vi "close.vi"(8 "error in":errorcluster, 11 "Sequencer Module runtime in":refnum<class "Sequencer Module runtime.lvclass">) -> (0 "error out":errorcluster)   [LabVIEW 2015, in "Sequencer Module runtime.lvclass"]
doc: "Provides an interface for terminating a module instance. While this interface performs no operations, a child should close and deallocate any open references or memory."
uses:
  Sequencer Module runtime.lvclass
  Sequencer Module runtime.lvclass/Sequencer Module runtime.ctl
  classes/Result Processor/Execution/ResultProcessor.lvclass
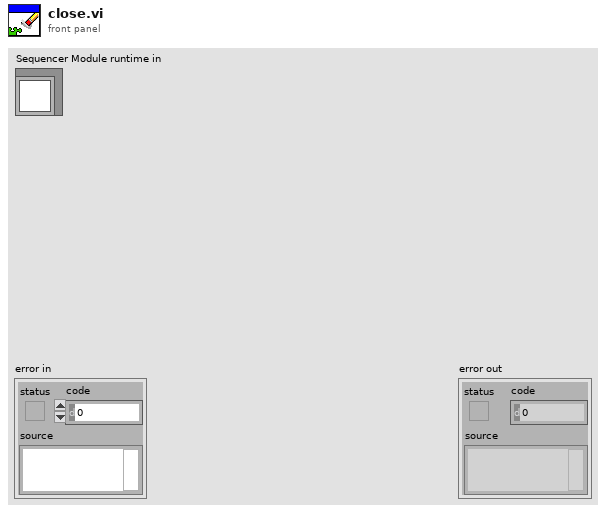
[diagram p1: front panel]
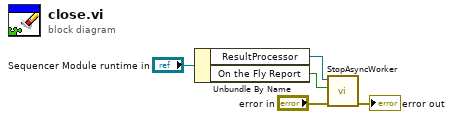
[diagram p0: block diagram]
diagram:
  n1 = Unbundle By Name("Sequencer Module runtime in") -> ("ResultProcessor"=w2:refnum<class "ResultProcessor.lvclass">, "On the Fly Report"=w1:bool)
  n2 = call "StopAsyncWorker.vi"("error in (no error)"="error in", "WaitOnAsync?"=w1, "ResultProcessor in"=w2) -> ("error out"=→"error out":errorcluster)  [unwired: 7 in, 1 out]
